vi "moveInParallelWay.vi"(7 "Game":refnum<class "Game.lvclass">, 8 "error in (no error)":errorcluster, 10 "Robot":refnum<class "Robot.lvclass">, 11 "MoveFromBallPlacementInterferenceSkill in":refnum<class "MoveFromBallPlacementInterferenceSkill.lvclass">) -> (0 "error out":errorcluster, 2 "finalPositionToGo":dbl[](array[numeric]), 3 "MoveFromBallPlacementInterferenceSkill out":refnum<class "MoveFromBallPlacementInterferenceSkill.lvclass">)   [LabVIEW 2020, in "MoveFromBallPlacementInterferenceSkill.lvclass"]
uses:
  MoveFromBallPlacementInterferenceSkill.lvclass
  Robot_class/Robot.lvclass
  C:/RoboIME/SSL_AI/Object_class/Object.lvclass
  Game_class/Game.lvclass
  Game_class/Game.lvclass/Game.ctl
  Object_class/Object.lvclass/Object.ctl
  <vilib>/Analysis/baseanly.llb/Real Dot Product.vi
  <vilib>/Analysis/baseanly.llb/Unit Vector (DBL).vi
  Object_class/Read position(x,y).vi
  Game_class/Read BallRef.vi
  Game_class/Read Referee.vi
  Ball_class/Ball.lvclass
  Referee_class/Referee.lvclass
  <vilib>/Analysis/NI_AALBase.lvlib
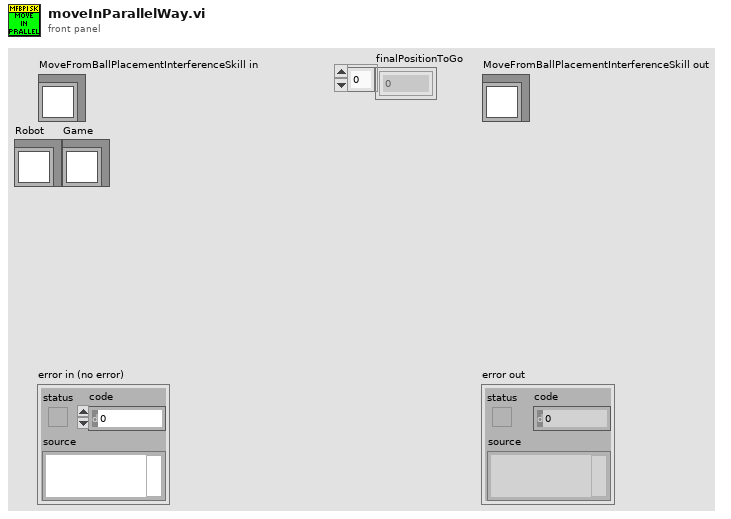
[diagram p1: front panel]
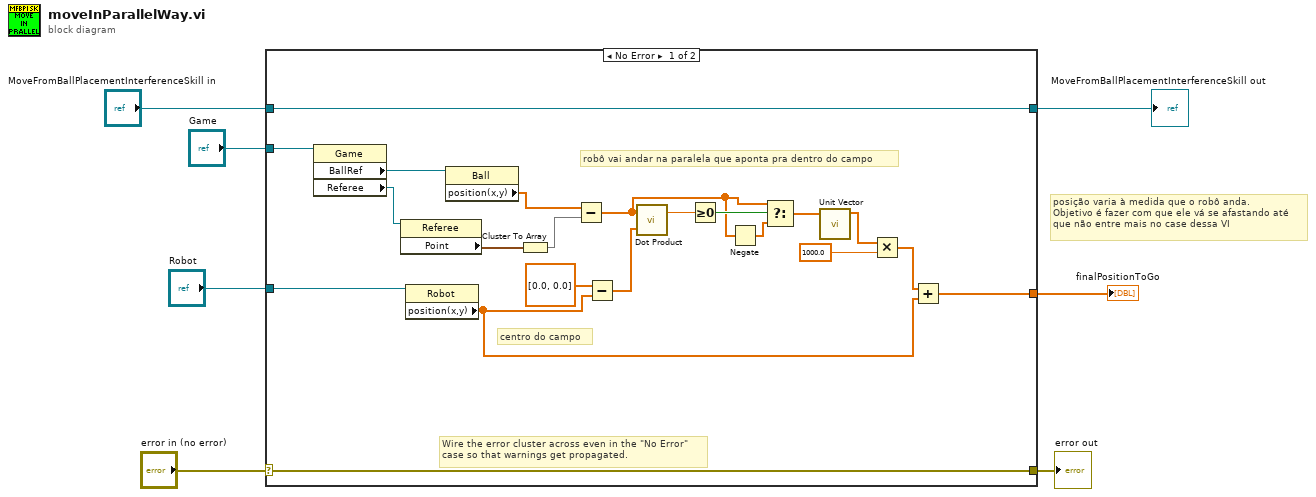
[diagram p0: block diagram]
diagram:
  # "posição varia à medida que o robô anda.\nObjetivo é fazer com que ele vá se afastando até\nque não entre mais no case dessa VI"
  n1 = case shown="No Error" "error in (no error)" {
    selector: "error in (no error)" -> [w27 w30]
    tunnel: [w27 w30] -> w6
    tunnel: [w28 w29] -> w4
    tunnel: "MoveFromBallPlacementInterferenceSkill in" -> [w28 w29]
    tunnel: "Game" -> [w26 _]
    tunnel: "Robot" -> [w20 _]
    tunnel: [w8 _] -> w1
    frame No Error {
      # "robô vai andar na paralela que aponta pra dentro do campo"
      # "centro do campo"
      # "Wire the error cluster across even in the \"No Error\"\ncase so that warnings get propagated."
      n2 = property class="Game"(reference=w26) -> ("BallRef"=w25:refnum<class "Ball.lvclass">, "Referee"=w24:refnum<class "Referee.lvclass">)  [unwired: 1 in, 2 out]
      n3 = property class="Referee"(reference=w24) -> ("Point"=w23:cluster{"x":sgl, "y":sgl})  [unwired: 1 in, 2 out]
      n4 = property class="Robot"(reference=w20) -> ("position(x,y)"=w12:dbl[])  [unwired: 1 in, 2 out]
      n5 = property class="Ball"(reference=w25) -> ("position(x,y)"=w22:dbl[])  [unwired: 1 in, 2 out]
      n6 = Cluster To Array(cluster=w23) -> (array=w21:sgl[])
      n7 = Subtract(x=w22, y=w21) -> (x-y=w15:dbl[])
      n8 = Subtract(x=dbl[] [0.0, 0.0], y=w12) -> (x-y=w18:dbl[])
      n9 = call-poly <vilib>:"Dot Product.vi"("Y Vector"=w18, "X Vector"=w15) -> ("X * Y"=w17:dbl)  [unwired: 1 out]
      n10 = Greater Or Equal To 0?(x=w17) -> (x >= 0?=w16:bool)
      n11 = Negate(x=w15) -> (-x=w14:dbl[])
      n12 = Select(t=w15, s=w16, f=w14) -> (s? t:f=w13:dbl[])
      n13 = call-poly <vilib>:"Unit Vector.vi"("Input Vector"=w13) -> ("Unit Vector"=w11:dbl[])  [unwired: 8 in, 2 out]
      n14 = Multiply(x=w11, y=1000.0) -> (x*y=w10:dbl[])
      n15 = Add(x=w10, y=w12) -> (x+y=w8:dbl[])
    }
    frame Error {
    }
  }
  "error out" <- w6
  "MoveFromBallPlacementInterferenceSkill out" <- w4
  "finalPositionToGo" <- w1
